vi "Detect QRCodes.vi"   [LabVIEW 2020, in "g_ar_toolkit.feature_detection.lvlib" / "QRDetector.lvclass"]
uses:
  QRDetector.lvclass
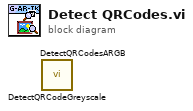
[diagram p0: block diagram]
diagram:
  n1 = call "DetectQRCodeGreyscale.vi"() -> ()  [unwired: 9 in, 3 out]
  n2 = call "DetectQRCodesARGB.vi"() -> ()  [unwired: 9 in, 3 out]
